vi "laserSetPower.vi"(8 "error in (no error)":errorcluster, 10 "Laser Power (mW)":dbl, 11 "VISA Refnum in":refnum<visa-resource-name>) -> (0 "error out":errorcluster, 3 "VISA Refnum out":refnum<visa-resource-name>)   [LabVIEW 2011]
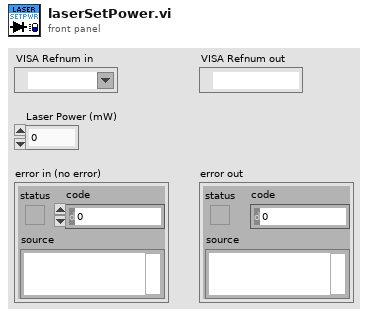
[diagram p1: front panel]
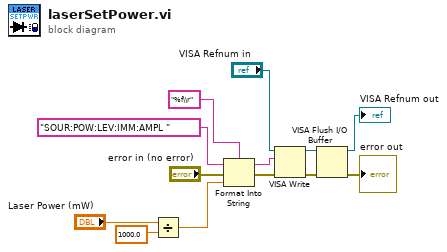
[diagram p0: block diagram]
diagram:
  n1 = Divide(x="Laser Power (mW)", y=1000.0) -> (x/y=w7:dbl)
  n2 = Format Into String(format string="%f\\r", initial string="SOUR:POW:LEV:IMM:AMPL " ("write buffer"), error in="error in (no error)", w7) -> (resulting string=w13:string, error out=w9:errorcluster)
  n3 = VISA Write(VISA resource name="VISA Refnum in", write buffer=w13, error in (no error)=w9) -> (VISA resource name out=w2:refnum<visa-resource-name>, error out=w1:errorcluster)  [unwired: 1 out]
  n4 = VISA Flush I/O Buffer(VISA resource name=w2, error in (no error)=w1) -> (VISA resource name out=→"VISA Refnum out":refnum<visa-resource-name>, error out=→"error out":errorcluster)  [unwired: 1 in]
